vi "Configure Dual Arbitrary Waveform.vi"(6 "Offset (0 V)":dbl, 7 "Enable Balancing (T: Enable)":bool=TRUE, 8 "error in (no error)":errorcluster, 9 "Gain Balancing Ratio (0)":dbl, 10 "Channel (1: 1)":i32(ring)=1 items=["1"=1, "2"=2], 11 "VISA resource name":refnum<visa-resource-name>) -> (0 "error out":errorcluster, 3 "VISA resource name out":refnum<visa-resource-name>)   [LabVIEW 2013, in "AWG.lvlib" / "Agilent 3352X Series.lvlib"]
doc: "Configurations for the balance of dual arbitrary waveforms."
uses:
  Agilent 3352X Series.lvlib
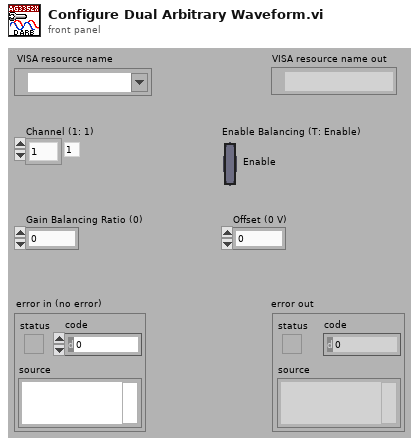
[diagram p1: front panel]
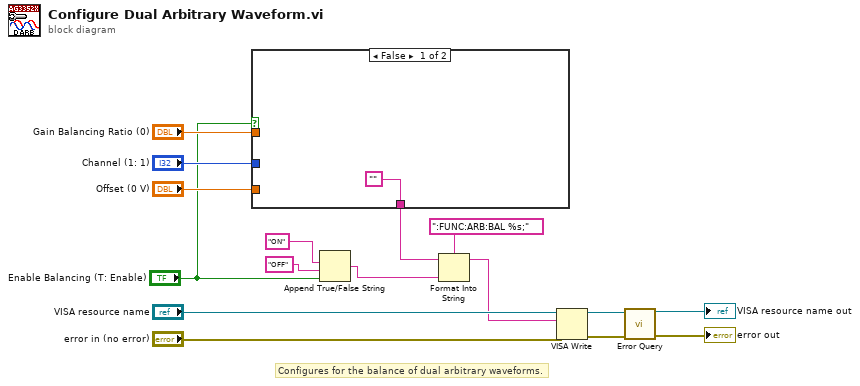
[diagram p0: block diagram]
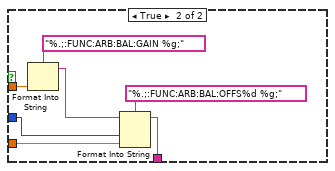
[diagram p2: hidden frame]
diagram:
  # "Configures for the balance of dual arbitrary waveforms."
  n1 = case shown="False" "Enable Balancing (T: Enable)" {
    tunnel: "Offset (0 V)" -> [_ w23]
    tunnel: "Gain Balancing Ratio (0)" -> [_ w22]
    tunnel: ["" ("Empty String Constant") w20] -> w3
    tunnel: "Channel (1: 1)" -> [_ w18]
    frame False {
    }
    frame True {
      n2 = Format Into String(format string="%.;:FUNC:ARB:BAL:GAIN %g;", w22) -> (resulting string=w19:string)  [unwired: 2 in, 1 out]
      n3 = Format Into String(format string="%.;:FUNC:ARB:BAL:OFFS%d %g;", initial string=w19, w18, w23) -> (resulting string=w20:string)  [unwired: 1 in, 1 out]
    }
  }
  n4 = Append True/False String(1:"Enable Balancing (T: Enable)", 2:"OFF" ("false string"), 3:"ON" ("true string")) -> (0:w5:string)  [unwired: 1 out]
  n5 = Format Into String(format string=":FUNC:ARB:BAL %s;", initial string=w3, w5) -> (resulting string=w2:string)  [unwired: 1 in, 1 out]
  n6 = VISA Write(VISA resource name="VISA resource name", write buffer=w2, error in (no error)="error in (no error)") -> (VISA resource name out=w12:refnum<visa-resource-name>, error out=w11:errorcluster)  [unwired: 1 out]
  n7 = call "Error Query.vi"("error in (no error)"=w11, "VISA resource name"=w12) -> ("error out"=→"error out":errorcluster, "VISA resource name out"=→"VISA resource name out":refnum<visa-resource-name>)  [unwired: 8 out]
